vi "Create Data File.vi"(8 "error in (no error)":errorcluster caption="错误输入（无错误）", 10 "Acquisition and Logging Configuration":T1={"Samples per Read"=100, "Number of Reads to Save"=20, "Number of Channels"=4, "Channel Scale Array"=[1.0, 1.0, 1.0, 1.0], "Channel Names"=[], "Trigger - RMS Value"=0.9999999999999994, "Trigger - Channel"=0, "Trigger - Time (Minute)"=10, "TDMS Properties"=[], "Data File Name"="cRIO_Data", "Date Rate"=20} caption="采集与记录配置" {"Date Rate" items=["51.200 kS/s (NI 9234)"=1, "25.600 kS/s (NI 9234)"=2, "17.067 kS/s (NI 9234)"=3, "12.80 kS/s (NI 9234)"=4, "10.240 kS/s (NI 9234)"=5, "8.533 kS/s (NI 9234)"=6, "7.314 kS/s (NI 9234)"=7, "6.400 kS/s (NI 9234)"=8, "5.689 kS/s (NI 9234)"=9, "5.120 kS/s (NI 9234)"=10, "4.654 kS/s (NI 9234)"=11, "4.267 kS/s (NI 9234)"=12, "3.938 kS/s (NI 9234)"=13, "3.657 kS/s (NI 9234)"=14, "3.413 kS/s (NI 9234)"=15, "3.200 kS/s (NI 9234)"=16, "3.012 kS/s (NI 9234)"=17, "2.845 kS/s (NI 9234)"=18, "2.695 kS/s (NI 9234)"=19, "2.560 kS/s (NI 9234)"=20, "2.438 kS/s (NI 9234)"=21, "2.328 kS/s (NI 9234)"=22, "2.226 kS/s (NI 9234)"=23, "2.133 kS/s (NI 9234)"=24, "2.048 kS/s (NI 9234)"=25, "1.969 kS/s (NI 9234)"=26, "1.896 kS/s (NI 9234)"=27, "1.829 kS/s (NI 9234)"=28, "1.765 kS/s (NI 9234)"=29, "1.707 kS/s (NI 9234)"=30, "1.652 kS/s (NI 9234)"=31]}) -> (0 "error out":errorcluster caption="错误输出", 3 "TDMS File Reference":refnum<k34> caption="TDMS文件引用")   [LabVIEW 2013]
doc: "读取DMA FIFO的波形数据。"
uses:
  controls/Acquisition and Logging Configuration.ctl
  controls/TDMS Properties.ctl
  <vilib>/LabVIEW Targets/FPGA/cRIO/shared/nicrio_ModuleControls/nicrio_cRIO-9234_DataRatesRing2.ctl
  Globals/Global - Configuration Options.vi
panel:
  # "通道"
  # "保存"
  # "采样"
  # "触发"
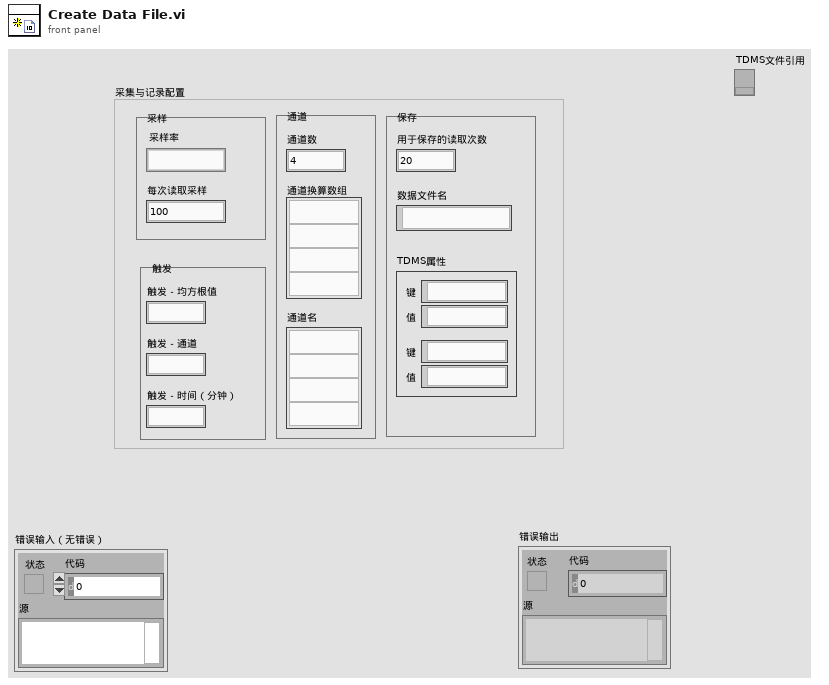
[diagram p1: front panel]
types:
  T1 = typedef "Acquisition and Logging Configuration.ctl" = cluster{"Samples per Read":i32, "Number of Reads to Save":i32, "Number of Channels":i32, "Channel Scale Array":fxp<+,24,12>[], "Channel Names":string[], "Trigger - RMS Value":dbl, "Trigger - Channel":i32, "Trigger - Time (Minute)":i32, "TDMS Properties":T2[], "Data File Name":string, "Date Rate":T3}
  T2 = typedef "TDMS Properties.ctl" = cluster{"Name":string, "Value":string}
  T3 = typedef "nicrio_cRIO-9234_DataRatesRing2.ctl" = u16
  T4 = enum16{"open", "open or create", "create or replace", "create", "open (read-only)"}
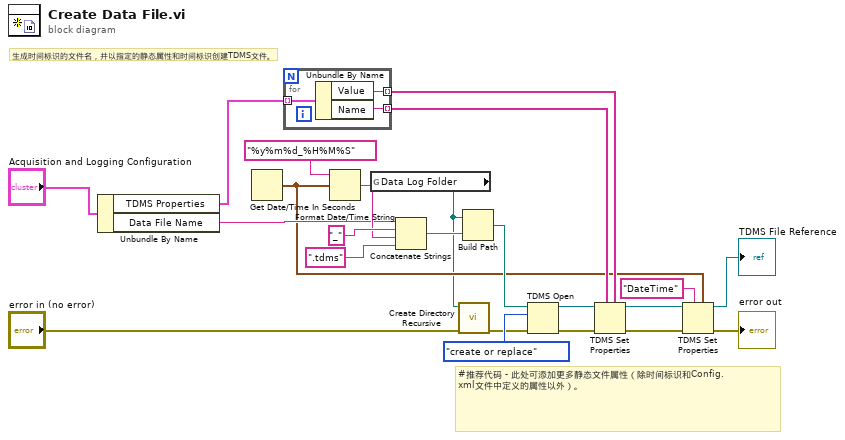
[diagram p0: block diagram]
diagram:
  # "生成时间标识的文件名，并以指定的静态属性和时间标识创建TDMS文件。"
  # "#推荐代码 - 此处可添加更多静态文件属性（除时间标识和Config.xml文件中定义的属性以外）。"
  n1 = Unbundle By Name("Acquisition and Logging Configuration") -> ("TDMS Properties"=w12:T2[], "Data File Name"=w18:string)
  n2 = Get Date/Time In Seconds() -> (seconds since 1Jan1904=w8:timestamp)
  n3 = for {
    tunnel: w12 -> [w26] mode=indexing
    tunnel: [w25] -> w11 mode=indexing
    tunnel: [w24] -> w10 mode=indexing
    n4 = Unbundle By Name(w26) -> ("Value"=w24:string, "Name"=w25:string)
  }
  n5 = Format Date/Time String(time format string (%c)="%y%m%d_%H%M%S", seconds (now)=w8) -> (date/time string=w22:string)  [unwired: 1 out]
  n6 = global read "Global - Configuration Options.vi" "Data Log Folder"() -> (w1:path)
  n7 = Concatenate Strings(w18, "_" ("string"), w22, ".tdms" ("string")) -> (w17:string)
  n8 = call <vilib>:"Create Directory Recursive.vi"("error in (no error)"="error in (no error)", "directory"=w1) -> ("error out"=w3:errorcluster)  [unwired: 3 in, 2 out]
  n9 = Build Path(base path=w1, name or relative path=w17) -> (appended path=w15:path)
  n10 = TDMS Open(8:w3, 10:T4."create or replace" ("operation (0:open)"), 11:w15) -> (0:w14:errorcluster, 3:w13:refnum<k34>)  [unwired: 4 in]
  n11 = TDMS Set Properties(5:w10, 7:w11, 8:w14, 11:w13) -> (0:w9:errorcluster, 3:w5:refnum<k34>)  [unwired: 2 in, 2 out]
  n12 = TDMS Set Properties(5:w8, 7:"DateTime" ("property names"), 8:w9, 11:w5) -> (0:→"error out":errorcluster, 3:→"TDMS File Reference":refnum<k34>)  [unwired: 2 in, 2 out]
